vi "_EnumEditor_BuildMenu.vi"(8 "error in (no error)":errorcluster, 10 "menu reference":refnum<k9>, 11 "_EnumEditor in":refnum<class "_EnumEditor.lvclass">) -> (0 "error out":errorcluster, 3 "_EnumEditor out":refnum<class "_EnumEditor.lvclass">)   [LabVIEW 2014, in "_EnumEditor.lvclass"]
uses:
  _EnumEditor.lvclass
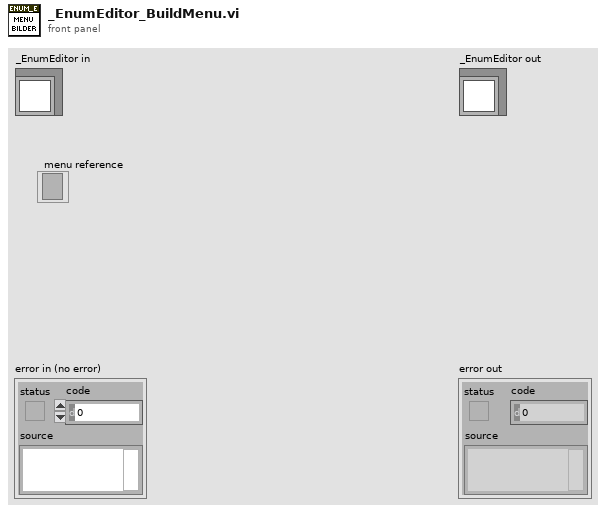
[diagram p1: front panel]
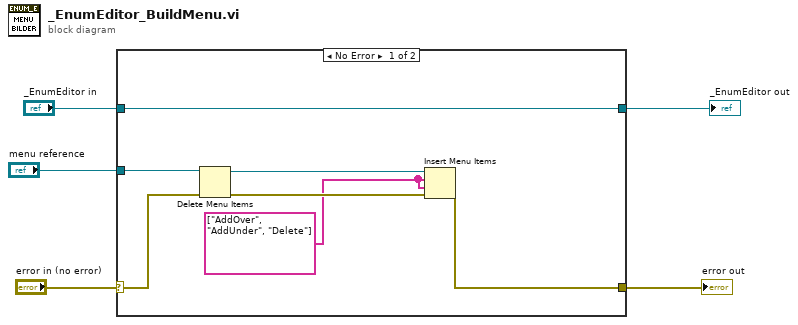
[diagram p0: block diagram]
diagram:
  n1 = case shown="No Error" "error in (no error)" {
    selector: "error in (no error)" -> [w7 w14]
    tunnel: [w9 w14] -> w4
    tunnel: [w12 w13] -> w2
    tunnel: "_EnumEditor in" -> [w12 w13]
    tunnel: "menu reference" -> [w10 _]
    frame No Error {
      w6 = string[] ["AddOver", "AddUnder", "Delete"]
      n2 = Delete Menu Items(6:w7, 9:w10) -> (0:w8:errorcluster, 3:w11:refnum<k9>)  [unwired: 2 in]
      n3 = Insert Menu Items(6:w8, 7:w6, 8:w6, 9:w11) -> (0:w9:errorcluster)  [unwired: 2 in, 2 out]
    }
    frame Error {
    }
  }
  "error out" <- w4
  "_EnumEditor out" <- w2
